vi "HFRR ADV v016 new software.vi"() -> ()   [LabVIEW 2025] (continued)
    n1463 = formula code="// Dynamic Parameterized Linear Interpolation Node\n// Inputs: vpp_val, voltages (Array), distances (Array)\n// Outputs: stroke\n\nint i = 0;\nint segments = 11; // 12 points make 11 interpolation segments\n\n// 1. Lower Boundary Clamp\nif (vpp_val <= voltages[0]) {\n    stroke = distances[0];\n}\n// 2. Upper Boundary Clamp\nelse if (vpp_val >= voltages[segments]) {\n    stroke = distances[segments];\n}\n// 3. Dynamic Segment Search Loop\nelse {\n    stroke = distances[0]; // Fallback baseline\n    for (i = 0; i < segments; i++) {\n        if (vpp_val >= voltages[i] && vpp_val <= voltages[i+1]) {\n            // Standard linear interpolation formula using array lookups\n            stroke = distances[i] + (vpp_val - voltages[i]) * (distances[i+1] - distances[i]) / (voltages[i+1] - voltages[i]);\n            break; // Segment found, safely exit the loop\n        }\n    }\n}"("vpp_val"=w1655, "voltages"="calibration values", "distances"="STROKE") -> ("stroke"=→"LVDT STROKE":dbl)
    n1464 = local read "Calibration Tare Value"() -> (w1659:dbl)
    n1465 = local read "Calibration Tare"() -> (w1657:bool)
    n1466 = Subtract(x=w1654, y=w1659) -> (x-y=→"LVDT STROKE  Calibration":dbl)
    n1467 = case shown="True" w1657 {
      selector: w1657 -> [_ w1665]
      tunnel: w1654 -> [_ w1666]
      frame False {
      }
      frame True {
        n1468 = Not(x=w1665) -> (.not. x?=w1664:bool)
        n1469 = local write "Calibration Tare"(w1664) -> ()
        "Calibration Tare Value" <- w1666
      }
    }
    n1470 = local read "Quit"() -> (w1663:bool)
  }
  n1471 = while {
    stop <- w1686 stop-if-true
    n1472 = call <vilib>:"High Resolution Polling Wait.vi"("seconds to wait"=0.02) -> ()  [unwired: 10 in, 1 out]
    n1473 = local read "Due read"() -> (w1684:string)
    n1474 = Spreadsheet String To Array(delimiter (Tab)=";", format string="", spreadsheet string=w1684, array type (2D Dbl)=string[] []) -> (array=w1681:string[])
    n1475 = Fract/Exp String To Number(string=w1681) -> (number=w1680:dbl[])  [unwired: 3 in, 1 out]
    n1476 = Index Array(array=w1680) -> (element #1=→"Sample Temperature":dbl, element #2=→"Target Sample Temperature":dbl, element #3=→"Current Duty Cycle":dbl, element #4=→"Ambient Temperature":dbl, element #5=→"Dac Status":dbl, element #6=→"Vpp":dbl, element #7=→"Active Error Code":dbl, element #8=→"Kp":dbl, element #9=→"Ki":dbl, element #10=→"Kd":dbl, element #11=→"SampleRaw":dbl, element #12=→"AmbRaw":dbl)  [unwired: 12 in]
    n1477 = local read "Quit"() -> (w1686:bool)
  }
  n1478 = while {
    shift-right: [w1700] -> w37
    shift-left: _ -> [w1691]
    shift-right: [w1699] -> w36
    shift-left: errorcluster {"status"=FALSE, "code"=0, "source"="Init"} ("error out") -> [w1693]
    tunnel: [w1688] -> w41
    tunnel: [w1698] -> _
    i -> [w1698]
    stop <- w1688 stop-if-true
    n1479 = local read "Com Port 2"() -> (w1692:refnum<visa-resource-name>)
    n1480 = local read "Port 2a"() -> (w1694:bool)
    n1481 = Unbundle(w1693) -> ("status"=→"Port 4":bool)  [unwired: 2 out]
    n1482 = call <vilib>:"High Resolution Polling Wait.vi"("seconds to wait"=0.02) -> ()  [unwired: 10 in, 1 out]
    n1483 = local read "Port 4"() -> (w1695:bool)
    n1484 = Not Equal?(x=w1692, y=w1691) -> (x != y?=w1690:bool)
    n1485 = Or(x=w1695, y=w1694) -> (x .or. y?=w1697:bool)
    n1486 = case shown="False" w1697 {
      frame False {
        w1703 = TRUE ("Visible")
        n1487 = property on="Port 2a" class="Bool (strict)"("Visible"=w1703) -> ()  [unwired: 2 in, 2 out]
        n1488 = property on="Port 4" class="Bool (strict)"("Visible"=w1703) -> ()  [unwired: 2 in, 2 out]
      }
      frame True {
        w1704 = TRUE ("Visible")
        n1489 = property on="Port 2a" class="Bool (strict)"("Visible"=w1704) -> ()  [unwired: 2 in, 2 out]
        n1490 = property on="Port 4" class="Bool (strict)"("Visible"=w1704) -> ()  [unwired: 2 in, 2 out]
      }
    }
    n1491 = case shown="True" w1690 {
      tunnel: [w1701 errorcluster {"status"=TRUE, "code"=0, "source"="Init"} ("error out")] -> w1689
      tunnel: w1693 -> [w1701 _]
      frame False {
      }
      frame True {
      }
    }
    n1492 = case shown="No Error" w1689 {
      selector: w1689 -> [w1717 w1748]
      tunnel: [w1710 w1753] -> w1700
      tunnel: [w1718 w1746] -> w1699
      tunnel: w1691 -> [w1719 w1751]
      frame No Error {
        n1493 = property class="Instr" props=["Serial Settings:Number of Bytes at Serial Port"](reference=w1719, error in=w1717) -> (reference out=w1711:refnum<visa-resource-name>, error out=w1716:errorcluster)  [unwired: 1 out]
        n1494 = while {
          tunnel: [w1727] -> w1712
          tunnel: [w1726] -> w1713
          tunnel: w1716 -> [w1725]
          tunnel: w1711 -> [w1724]
          tunnel: [w1723] -> _
          i -> [w1723]
          stop <- TRUE stop-if-true
          n1495 = property class="Instr" props=["Serial Settings:Number of Bytes at Serial Port"](reference=w1724, error in=w1725) -> (reference out=w1729:refnum<visa-resource-name>, error out=w1728:errorcluster)  [unwired: 1 out]
          n1496 = VISA Read(VISA resource name=w1729, byte count=u32 1000, error in (no error)=w1728) -> (VISA resource name out=w1726:refnum<visa-resource-name>, read buffer=→"Due read":string, error out=w1727:errorcluster)  [unwired: 1 out]
        }
        n1497 = local read "Command"() -> (w1709:string)
        n1498 = call <vilib>:"Trim Whitespace.vi"("string"=w1709) -> ("trimmed string"=w1708:string)  [unwired: 1 in]
        n1499 = Not Equal?(x=w1708, y="") -> (x != y?=w1714:bool)
        n1500 = VISA Flush I/O Buffer(VISA resource name=w1713) -> (VISA resource name out=w1706:refnum<visa-resource-name>, error out=→"error out 10":errorcluster)  [unwired: 2 in]
        n1501 = case shown="True" w1714 {
          tunnel: w1706 -> [w1731 w1736]
          tunnel: [w1731 w1740] -> w1710
          tunnel: w1712 -> [w1730 w1735]
          tunnel: [w1730 w1738] -> w1718
          tunnel: w1708 -> [_ w1734]
          tunnel: [_ w1737] -> _
          frame False {
            # "DATA  WRITE LOOP"
          }
          frame True {
            n1502 = Concatenate Strings(w1734, "\r\n") -> (w1733:string)
            n1503 = VISA Write(VISA resource name=w1736, write buffer=w1733, error in (no error)=w1735) -> (VISA resource name out=w1740:refnum<visa-resource-name>, return count=w1737:u32, error out=w1739:errorcluster)
            n1504 = flat-sequence {
              tunnel: w1739 -> [w1742]
              tunnel: [w1742] -> w1738
              frame #0 {
                n1505 = local write "Command"("" ("Command")) -> ()
                n1506 = Wait (ms)(milliseconds to wait=u32 5) -> ()  [unwired: 1 out]
              }
            }
          }
        }
        "Port 2a" <- TRUE ("Port 2a")
      }
      frame Error {
        w1759 = u16 0 items=["None", "XON/XOFF", "RTS/CTS", "XON/XOFF & RTS/CTS", "DTR/DSR", "XON/XOFF & DTR/DSR"] ("flow control (0:none)  2")
        w1757 = u16 10 items=["1.0"=10, "1.5"=15, "2.0"=20] ("stop bits 2")
        w1755 = u16 0 items=["None", "Odd", "Even", "Mark", "Space"] ("parity 2")
        w1756 = u32 10000  # timeout (10sec)
        n1507 = VISA Clear(VISA resource name=w1751, error in (no error)=w1748) -> (VISA resource name out=w1750:refnum<visa-resource-name>, error out=w1749:errorcluster)
        n1508 = VISA Close(VISA resource name=w1750, error in (no error)=w1749) -> (error out=w1752:errorcluster)
        n1509 = call <vilib>:"Clear Errors.vi"("error in (no error)"=w1752) -> ()  [unwired: 5 in, 2 out]
        n1510 = local write "Port 2a"(FALSE ("Port 2a")) -> ()
        n1511 = local read "Com Port 2"() -> (w1745:refnum<visa-resource-name>)
        "visa due" <- w1745
        n1512 = call-poly "VISA Configure Serial Port"("VISA resource name"=w1745, "timeout (10sec)"=w1756, "baud rate (9600)"=u32 250000 ("baud rate  2"), "data bits (8)"=u16 8 ("data bits  2"), "parity (0:none)"=w1755, "stop bits (10: 1 bit)"=w1757, "flow control (0:none)"=w1759) -> ("VISA resource name out"=w1760:refnum<visa-resource-name>, "error out"=w1761:errorcluster)  [unwired: 7 in]
        n1513 = flat-sequence {
          tunnel: w1760 -> [w1763]
          tunnel: w1761 -> [w1762]
          tunnel: [w1763] -> w1753
          tunnel: [w1762] -> w1746
          frame #0 {
            n1514 = Wait (ms)(milliseconds to wait=u32 50) -> ()  [unwired: 1 out]
          }
        }
        "Residual Due" <- ""
        "Port 2 Error" <- w1746
      }
    }
    n1515 = local read "Quit"() -> (w1688:bool)
    "Error Due" <- w1693
  }
  n1516 = local write "FRICVALZ"(0.0 ("FRICVALZ")) -> ()
  n1517 = property on="RUN" class="Bool (strict)"("Visible"=TRUE) -> ()  [unwired: 2 in, 2 out]
  n1518 = while {
    tunnel: [w1780] -> _
    tunnel: [w1765] -> w54
    i -> [w1780]
    stop <- w1765 stop-if-true
    n1519 = local read "conststatus"() -> (w1769:dbl)
    n1520 = local read "Main Tab"() -> (w1767:T2)
    n1521 = local read "EDIT"() -> (w1786:bool)
    n1522 = local read "Rate"() -> (w1785:dbl)
    n1523 = case shown="True" w1786 {
      tunnel: [FALSE TRUE] -> w1772
      frame False {
      }
      frame True {
      }
    }
    n1524 = property on="Time slide" class="Slide (strict)"("Scale.Range:Maximum"=2500.0) -> ()  [unwired: 2 in, 2 out]
    n1525 = Equal?(x=w1767, y=T27."About" ("Main Tab")) -> (x = y?=w1778:bool)
    n1526 = Equal?(x=w1769, y=0.0) -> (x = y?=w1770:bool)
    n1527 = Divide(x=1.0, y=w1785) -> (x/y=w1781:dbl)
    "Time 2" <- w1781
    n1528 = case shown="True" w1770 {
      frame False {
      }
      frame True {
        # "C:\\WinDucom\\calibrate WO 2391.dcf"
        n1529 = local write "Lan flag"(22) -> ()
        n1530 = local write "conststatus"(10.0 ("rpm value : 2")) -> ()
        n1531 = String To Path(string="C:\\LAB-IQ\\calibrate WO 2465.dcf") -> (path=w1792:path)
        n1532 = Open/Create/Replace File "Open File"(file path (use dialog)=w1792) -> (refnum out=w1790:refnum<file>)  [unwired: 5 in, 2 out]
        n1533 = for {
          N: 23 -> [_]
          tunnel: w1790 -> [w1801]
          i -> [w1795]
          (unwired) TRUE ("line mode (F)")
          n1534 = Read from Text File "Read File"(file (use dialog)=w1801) -> (text=w1800:string)  [unwired: 3 in, 3 out]
          n1535 = Match Pattern(string=w1800, regular expression="]") -> (after substring=w1798:string)  [unwired: 1 in, 3 out]
          n1536 = String Subset(string=w1800, offset (0)=5, length (rest)=10 ("length (rest)")) -> (substring=w1793:string)
          n1537 = Fract/Exp String To Number(string=w1793) -> (number=w1794:dbl)  [unwired: 3 in, 1 out]
          n1538 = Match Pattern(string=w1798, regular expression="-") -> (before substring=w1796:string)  [unwired: 1 in, 3 out]
          n1539 = case shown="19" w1795 {
            tunnel: w1794 -> [w1804 w1805 w1806 w1807 _ _ _ w1812 w1813 _ w1814 w1815 w1816 w1817 w1818 w1819 _ w1820 w1821 _ _ _ _ _]
            tunnel: w1796 -> [_ _ _ _ w1808 w1809 w1810 _ _ _ _ _ _ _ _ _ _ _ _ w1822 w1823 w1824 w1825 _]
            frame 0 {
              n1540 = local write "FRIC. FORCE :"(w1804) -> ()
            }
            frame 1 {
              n1541 = local write "TEMPERATURE :"(w1805) -> ()
            }
            frame 2 {
              n1542 = local write "HUMIDITY:"(w1806) -> ()
            }
            frame 3 {
              n1543 = local write "AIR TEMPERATURE :"(w1807) -> ()
            }
            frame 4 {
              n1544 = local write "Com Port 1"(w1808) -> ()
            }
            frame 5 {
              n1545 = local write "Com Port 2"(w1809) -> ()
              n1546 = local write "visa due"(w1809) -> ()
            }
            frame 6 {
              n1547 = String To Path(string=w1810) -> (path=w1811:path)
              n1548 = local write "File Path"(w1811) -> ()
              "String" <- w1810
            }
            frame 7 {
              n1549 = local write "DISPLACEMENT :"(w1812) -> ()
            }
            frame 8 {
              n1550 = local write "STROKE GAIN :"(w1813) -> ()
            }
            frame 9 {
            }
            frame 10 {
              n1551 = local write "Language Selection"(w1814) -> ()
            }
            frame 11 {
              n1552 = local write "CH-POWER +"(w1815) -> ()
            }
            frame 12 {
              n1553 = local write "CH-POWER -"(w1816) -> ()
            }
            frame 13 {
              n1554 = local write "CH-HEATER"(w1817) -> ()
            }
            frame 14 {
              n1555 = local write "CH-HUMIDITY WET"(w1818) -> ()
            }
            frame 15 {
              n1556 = local write "CH-HUMIDITY DRY"(w1819) -> ()
            }
            frame 16 {
            }
            frame 17 {
              n1557 = local write "AIR TEMP INTERCEPT:"(w1820) -> ()
            }
            frame 18 {
              n1558 = local write "TEMP INTERCEPT:"(w1821) -> ()
            }
            frame 21 {
              n1559 = local write "S.NO"(w1822) -> ()
            }
            frame 22 {
              n1560 = local write "Com Port 3"(w1823) -> ()
            }
            frame 20 {
              n1561 = local write "Camera Port :"(w1824) -> ()
            }
            frame 19 {
              n1562 = local write "C3 :"(w1825) -> ()
            }
            frame 23, Default {
            }
          }
        }
      }
    }
    n1563 = Select(t=u32 2500 ("milliseconds to wait"), s=w1778, f=u32 500 ("milliseconds to wait")) -> (s? t:f=w1776:u32)
    n1564 = Multiply(x=w1781, y=w1776) -> (x*y=w1783:dbl)
    n1565 = property on="Time slide" class="Slide (strict)"("Visible"=w1772) -> ()  [unwired: 2 in, 2 out]
    n1566 = call "Elapsed Time2"("Time Target (s)"=w1783, "Auto Reset"=TRUE) -> ("Time has Elapsed"=w1773:bool)  [unwired: 10 in, 7 out]
    n1567 = case shown="True" w1773 {
      frame False {
      }
      frame True {
        n1568 = stacked-sequence {
          frame #0 {
            # "DATA PROCESSING"
            # "115 mV/N"
            n1569 = local read "Sample Temperature"() -> (w1828:dbl)
            n1570 = local read "RH Numeric:"() -> (w1835:dbl)
            n1571 = local read "HUMIDITY:"() -> (w1836:dbl)
            n1572 = local read "FRICVALZ"() -> (w1847:dbl)
            n1573 = local read "Friction"() -> (w1831:dbl)
            n1574 = Multiply(x=w1835, y=w1836) -> (x*y=→"Humidity ( %RH )" →"Hum" →"Hum 2":dbl)
            n1575 = call <vilib>:"Mean PtByPt.vi"("x"=w1828, "sample length"=100) -> ("mean"=w1827:dbl)  [unwired: 2 in, 1 out]
            "TEMP 2" <- w1827
            "TEMP 3" <- w1827
            n1576 = Subtract(x=w1831, y=w1847) -> (x-y=w1842:dbl)
            "FF 2" <- w1842
            "FF 4" <- w1842
            n1577 = local read "Ambient Temperature"() -> (→"AIR TEMP":dbl)
            n1578 = local read "TEMP"() -> (w1846:dbl)
            n1579 = local write "FF 3"(w1842) -> ()
            n1580 = Compound Arithmetic op=OR("FRICVALZ 4", "FRICVALZ 3", "FRICVALZ 2") -> (w1838:bool)
            n1581 = case shown="True" w1838 {
              tunnel: w1831 -> [_ w1853]
              frame False {
              }
              frame True {
                w1852 = FALSE ("FRICVALZ")
                n1582 = local write "FRICVALZ 3"(w1852) -> ()
                n1583 = local write "FRICVALZ 2"(w1852) -> ()
                n1584 = local write "FRICVALZ 4"(w1852) -> ()
                "FRICVALZ" <- w1853
              }
            }
            n1585 = Not A Number/Path/Refnum?(number/path/refnum=w1846) -> (NaN/Path/Refnum?=w1845:bool)
            n1586 = Not A Number/Path/Refnum?(number/path/refnum=w1842) -> (NaN/Path/Refnum?=w1844:bool)
            n1587 = Divide(x=w1842, y=1.96) -> (x/y=w1839:dbl)
            n1588 = Compound Arithmetic op=OR(w1845, w1844) -> (w1843:bool)
            n1589 = Not A Number/Path/Refnum?(number/path/refnum=w1839) -> (NaN/Path/Refnum?=w1840:bool)
            n1590 = case shown="True" w1843 {
              frame False {
              }
              frame True {
                n1591 = local write "TEMP"(0.0 ("TEMP")) -> ()
                n1592 = local write "FF 2"(0.0 ("FF 2")) -> ()
                n1593 = local write "reinit"(TRUE ("reinit")) -> ()
              }
            }
            n1594 = local write "TEMP"(w1827) -> ()
            n1595 = Select(t=0.0, s=w1840, f=w1839) -> (s? t:f=w1830:dbl)
            "COF 2" <- w1830
            n1596 = local write "COF 3"(w1830) -> ()
          }
        }
      }
    }
    n1597 = Wait (ms)(milliseconds to wait=u32 50) -> ()  [unwired: 1 out]
    n1598 = local read "Quit"() -> (w1765:bool)
    "Rate" <- 2500.0 ("No of Samples")
  }
  n1599 = while {
    tunnel: w57 -> [_]
    tunnel: [w1880] -> _
    tunnel: [w1856] -> w56
    i -> [w1880]
    stop <- w1856 stop-if-true
    # "C:\\LAB-IQ-NXT\\Scar View.exe"
    n1600 = local read "OK Button 16"() -> (w1869:bool)
    n1601 = local read "Main Tab"() -> (w1862:T2)
    n1602 = local read "service 3"() -> (w1863:bool)
    n1603 = local read "OPEN 6"() -> (w1865:bool)
    n1604 = local read "EDIT 2"() -> (w1867:bool)
    n1605 = flat-sequence {
      frame #0 {
        n1606 = local read "SAVE 2"() -> (w2482:bool)
        n1607 = stacked-sequence {
          frame #0 {
            n1608 = local read "EDIT"() -> (w2536:bool)
            n1609 = case shown="True" w2536 {
              tunnel: [u8 2 ("Disabled") u8 0 ("Disabled")] -> _
              frame False {
                w2538 = FALSE
                n1610 = local write "Password"("") -> ()
                n1611 = property on="SrvM CP" class="Bool (strict)"("Visible"=w2538) -> ()  [unwired: 2 in, 2 out]
                n1612 = property on="message" class="Str"("Visible"=w2538) -> ()  [unwired: 2 in, 2 out]
                n1613 = local write "x = y?"(w2538) -> ()
                n1614 = property on="Password" class="Str"("Visible"=w2538) -> ()  [unwired: 2 in, 2 out]
                n1615 = property on="ENTER THE NEW PASSWORD" class="Str"("Visible"=w2538) -> ()  [unwired: 2 in, 2 out]
                n1616 = property on="ENTER CURRENT PASSWORD" class="Str"("Visible"=w2538) -> ()  [unwired: 2 in, 2 out]
                n1617 = local write "SrvM CP"(w2538) -> ()
              }
              frame True {
                w2541 = TRUE
                n1618 = property on="SrvM CP" class="Bool (strict)"("Visible"=w2541) -> ()  [unwired: 2 in, 2 out]
                n1619 = property on="Password" class="Str"("Visible"=w2541) -> ()  [unwired: 2 in, 2 out]
              }
            }
            "dipl pwd" <- "@143$\n" ("dipl pwd")
          }
          frame #1 {
            # "Gain password"
            n1620 = String To Byte Array(string="ENTER CURRENT PASSWORD") -> (unsigned byte array=w2546:u8[])
            n1621 = Search 1D Array(1D array=w2546, element=u8 10) -> (index of element=w2549:i32)  [unwired: 1 in]
            n1622 = Index Array(array=w2546, index=w2549) -> (element=w2545:u8)
            n1623 = Equal?(x=w2545, y=10) -> (x = y?=w2543:bool)
            n1624 = case shown="True" w2543 {
              frame False {
                n1625 = property on="ENTER THE NEW PASSWORD" class="Str"("Visible"=FALSE) -> ()  [unwired: 2 in, 2 out]
              }
              frame True {
                # "password"
                # "change password logic"
                n1626 = local read "ENTER CURRENT PASSWORD"() -> (w2562:string)
                n1627 = local read "dipl pwd"() -> (w2556:string)
                n1628 = String To Byte Array(string=w2562) -> (unsigned byte array=w2564:u8[])
                n1629 = String To Byte Array(string=w2556) -> (unsigned byte array=w2557:u8[])
                n1630 = Array Size(array=w2564) -> (size(s)=w2561:i32)
                n1631 = Array Size(array=w2557) -> (size(s)=w2559:i32)
                n1632 = for {
                  N: w2561 -> [_]
                  tunnel: w2564 -> [w2588]
                  tunnel: [w2586] -> w2565 mode=indexing
                  tunnel: w2561 -> [w2580]
                  i -> [w2581]
                  n1633 = Decrement(x=w2580) -> (x-1=w2578:i32)
                  n1634 = Equal?(x=w2581, y=w2578) -> (x = y?=w2579:bool)
                  n1635 = Index Array(array=w2588, index=w2581) -> (element=w2582:u8)
                  n1636 = Number To Decimal String(number=w2582) -> (decimal integer string=w2587:string)  [unwired: 1 in]
                  n1637 = Select(t="", s=w2579, f="\r") -> (s? t:f=w2584:string)
                  n1638 = Concatenate Strings(w2587, w2584) -> (w2586:string)
                }
                n1639 = for {
                  N: w2559 -> [_]
                  tunnel: w2557 -> [w2576]
                  tunnel: [w2574] -> w2558 mode=indexing
                  tunnel: w2559 -> [w2571]
                  i -> [w2572]
                  n1640 = Decrement(x=w2571) -> (x-1=w2570:i32)
                  n1641 = Equal?(x=w2572, y=w2570) -> (x = y?=w2569:bool)
                  n1642 = Index Array(array=w2576, index=w2572) -> (element=w2575:u8)
                  n1643 = Number To Decimal String(number=w2575) -> (decimal integer string=w2573:string)  [unwired: 1 in]
                  n1644 = Select(t="", s=w2569, f="\r") -> (s? t:f=w2566:string)
                  n1645 = Concatenate Strings(w2573, w2566) -> (w2574:string)
                }
                n1646 = local read "string"() -> (w2563:string)
                n1647 = Concatenate Strings(w2558) -> (w2552:string)
                n1648 = Concatenate Strings(w2563) -> (w2560:string)
                n1649 = Concatenate Strings(w2565) -> (w2553:string)
                n1650 = Equal?(x=w2553, y=w2560) -> (x = y?=w2555:bool)
                n1651 = Equal?(x=w2553, y=w2552) -> (x = y?=w2551:bool)
                n1652 = Or(x=w2555, y=w2551) -> (x .or. y?=w2554:bool)
                n1653 = case shown="True" w2554 {
                  frame False {
                  }
                  frame True {
                    n1654 = property on="ENTER THE NEW PASSWORD" class="Str"("Visible"=TRUE) -> ()  [unwired: 2 in, 2 out]
                  }
                }
              }
            }
          }
          frame #2 {
            n1655 = String To Byte Array(string="ENTER THE NEW PASSWORD") -> (unsigned byte array=w2591:u8[])
            n1656 = Search 1D Array(1D array=w2591, element=u8 10) -> (index of element=w2595:i32)  [unwired: 1 in]
            n1657 = Index Array(array=w2591, index=w2595) -> (element=w2593:u8)
            n1658 = Equal?(x=w2593, y=10) -> (x = y?=w2590:bool)
            n1659 = case shown="False" w2590 {
              frame False {
              }
              frame True {
                n1660 = local write "EDIT"(FALSE) -> ()
                n1661 = local write "SrvM CP"(FALSE) -> ()
                n1662 = local read "ENTER THE NEW PASSWORD"() -> (w2598:string)
                n1663 = String To Byte Array(string=w2598) -> (unsigned byte array=w2603:u8[])
                n1664 = Array Size(array=w2603) -> (size(s)=w2600:i32)
                n1665 = for {
                  N: w2600 -> [_]
                  tunnel: w2603 -> [w2616]
                  tunnel: [w2613] -> w2605 mode=indexing
                  tunnel: w2600 -> [w2608]
                  i -> [w2606]
                  n1666 = Decrement(x=w2608) -> (x-1=w2609:i32)
                  n1667 = Equal?(x=w2606, y=w2609) -> (x = y?=w2610:bool)
                  n1668 = Index Array(array=w2616, index=w2606) -> (element=w2615:u8)
                  n1669 = Number To Decimal String(number=w2615) -> (decimal integer string=w2614:string)  [unwired: 1 in]
                  n1670 = Select(t="", s=w2610, f="\r") -> (s? t:f=w2607:string)
                  n1671 = Concatenate Strings(w2614, w2607) -> (w2613:string)
                }
                n1672 = local read "file path"() -> (w2597:path)
                n1673 = Concatenate Strings(w2605) -> (w2599:string)
                n1674 = Delete(path (use dialog)=w2597) -> (deleted path=w2601:path)  [unwired: 4 in, 2 out]
                n1675 = call <vilib>:"Write Characters To File.vi"("append to file? (new file:F)"=FALSE, "character string"=w2599, "file path (dialog if empty)"=w2601) -> ()  [unwired: 2 in, 1 out]
              }
            }
          }
          frame #3 {
            n1676 = case shown="True" "SrvM CP" {
              frame False {
                w2619 = ""
                n1677 = local write "ENTER CURRENT PASSWORD"(w2619) -> ()
                n1678 = local write "ENTER THE NEW PASSWORD"(w2619) -> ()
                n1679 = property on="ENTER CURRENT PASSWORD" class="Str"("Visible"=FALSE) -> ()  [unwired: 2 in, 2 out]
              }
              frame True {
                n1680 = property on="ENTER THE NEW PASSWORD" class="Str"() -> ("Visible"=w2620:bool)  [unwired: 2 in, 2 out]
                n1681 = Not(x=w2620) -> (.not. x?=w2621:bool)
                n1682 = property on="ENTER CURRENT PASSWORD" class="Str"("Visible"=w2621) -> ()  [unwired: 2 in, 2 out]
              }
            }
          }
          frame #4 {
            n1683 = String To Byte Array(string="Password") -> (unsigned byte array=w2628:u8[])
            n1684 = Search 1D Array(1D array=w2628, element=u8 10) -> (index of element=w2626:i32)  [unwired: 1 in]
            n1685 = Index Array(array=w2628, index=w2626) -> (element=w2627:u8)
            n1686 = Equal?(x=w2627, y=10) -> (x = y?=w2623:bool)
            n1687 = case shown="True" w2623 {
              frame False {
              }
              frame True {
                # "password"
                # "password"
                n1688 = local read "Password"() -> (w2641:string)
                n1689 = String To Byte Array(string=w2641) -> (unsigned byte array=w2644:u8[])
                n1690 = String To Byte Array(string="@143$\n") -> (unsigned byte array=w2630:u8[])
                n1691 = Array Size(array=w2644) -> (size(s)=w2639:i32)
                n1692 = Array Size(array=w2630) -> (size(s)=w2635:i32)
                n1693 = for {
                  N: w2639 -> [_]
                  tunnel: w2644 -> [w2678]
                  tunnel: [w2676] -> w2645 mode=indexing
                  tunnel: w2639 -> [w2673]
                  i -> [w2674]
                  n1694 = Decrement(x=w2673) -> (x-1=w2672:i32)
                  n1695 = Index Array(array=w2678, index=w2674) -> (element=w2677:u8)
                  n1696 = Equal?(x=w2674, y=w2672) -> (x = y?=w2671:bool)
                  n1697 = Number To Decimal String(number=w2677) -> (decimal integer string=w2675:string)  [unwired: 1 in]
                  n1698 = Select(t="", s=w2671, f="\r") -> (s? t:f=w2668:string)
                  n1699 = Concatenate Strings(w2675, w2668) -> (w2676:string)
                }
                n1700 = for {
                  N: w2635 -> [_]
                  tunnel: w2630 -> [w2689]
                  tunnel: [w2687] -> w2633 mode=indexing
                  tunnel: w2635 -> [w2684]
                  i -> [w2685]
                  n1701 = Decrement(x=w2684) -> (x-1=w2683:i32)
                  n1702 = Index Array(array=w2689, index=w2685) -> (element=w2688:u8)
                  n1703 = Equal?(x=w2685, y=w2683) -> (x = y?=w2682:bool)
                  n1704 = Number To Decimal String(number=w2688) -> (decimal integer string=w2686:string)  [unwired: 1 in]
                  n1705 = Select(t="", s=w2682, f="\r") -> (s? t:f=w2679:string)
                  n1706 = Concatenate Strings(w2686, w2679) -> (w2687:string)
                }
                n1707 = local read "file path"() -> (w2629:path)
                n1708 = call <vilib>:"Read Characters From File.vi"("file path (dialog if empty)"=w2629) -> ("character string"=w2643:string)  [unwired: 5 in, 3 out]
                "string" <- w2643
                n1709 = flat-sequence {
                  tunnel: [w2646] -> w2640
                  frame #0 {
                    w2646 = ""
                    n1710 = local write "Password"(w2646) -> ()
                  }
                }
                n1711 = Concatenate Strings(w2633) -> (w2634:string)
                n1712 = Concatenate Strings(w2643) -> (w2642:string)
                n1713 = Concatenate Strings(w2645) -> (w2637:string)
                n1714 = Equal?(x=w2637, y=w2642) -> (x = y?=w2632:bool)
                n1715 = Equal?(x=w2637, y=w2634) -> (x = y?=w2638:bool)
                n1716 = Or(x=w2632, y=w2638) -> (x .or. y?=w2631:bool)
                "x = y?" <- w2631
                n1717 = case shown="True" w2631 {
                  selector: w2631 -> [w2648 _]
                  tunnel: w2640 -> [_ _]
                  frame False {
                    n1718 = And(x=w2648, y=TRUE ("Visible")) -> (x .and. y?=w2649:bool)
                    n1719 = property on="message" class="Str"("Visible"=w2649) -> ()  [unwired: 2 in, 2 out]
                  }
                  frame True {
                    n1720 = control-ref of="This VI"() -> (w2660:refnum<vi>)
                    n1721 = property class="VI"(reference=w2660) -> (reference out=w2651:refnum<vi>, error out=w2655:errorcluster, "Panel"=w2659:refnum<vi>)  [unwired: 1 in]
                    n1722 = property on="message" class="Str"("Visible"=FALSE) -> ()  [unwired: 2 in, 2 out]
                    n1723 = property class="Pnl"(reference=w2659, error in=w2655) -> (reference out=w2653:refnum<vi>, error out=w2656:errorcluster, "Panes[]"=w2658:refnum<vi>[])
                    n1724 = for {
                      tunnel: w2658 -> [w2667] mode=indexing
                      tunnel: T21."Always On" ("Horizontal Scrollbar Visibility") -> [w2666]
                      tunnel: w2656 -> [w2663]
                      tunnel: [w2662] -> w2654
                      n1725 = property class="Pane"(reference=w2667, error in=w2663, "HorizScrollbarVisibility"=w2666) -> (reference out=w2664:refnum<vi>, error out=w2665:errorcluster)
                      n1726 = Close Reference(reference=w2664, error in (no error)=w2665) -> (error out=w2662:errorcluster)
                    }
                    n1727 = Close Reference(reference=w2653, error in (no error)=w2654) -> (error out=w2652:errorcluster)
                    n1728 = Close Reference(reference=w2651, error in (no error)=w2652) -> (error out=→"error out 6":errorcluster)
                  }
                }
              }
            }
          }
        }
        n1729 = local read "x = y?"() -> (w2488:bool)
        n1730 = local read "HUMIDITY: 2"() -> (w2490:dbl)
        n1731 = local read "HUMIDITY:"() -> (w2489:dbl)
        n1732 = property on="Port 2 Error" class="Clust (strict)"("Visible"="EDIT") -> ()  [unwired: 2 in, 2 out]
        n1733 = property on="Port 1 Error" class="Clust (strict)"("Visible"="EDIT") -> ()  [unwired: 2 in, 2 out]
        n1734 = case shown="True" "SrvM CP 2" {
          frame False {
          }
          frame True {
            n1735 = local write "SrvM CP 2"(FALSE ("SrvM CP 2")) -> ()
            n1736 = local read "HUMIDITY: 2"() -> (w2529:dbl)
            n1737 = local read "TEMP INTERCEPT: 2"() -> (w2528:dbl)
            n1738 = local read "DISPLACEMENT : 4"() -> (w2532:dbl)
            n1739 = local read "TEMPERATURE : 2"() -> (w2531:dbl)
            n1740 = local read "STROKE GAIN : 2"() -> (w2533:dbl)
            n1741 = local read "FRIC. FORCE : 2"() -> (w2534:dbl)
            n1742 = local read "AIR TEMP INTERCEPT: 2"() -> (w2527:dbl)
            n1743 = local read "AIR TEMPERATURE : 2"() -> (w2530:dbl)
            n1744 = local write "HUMIDITY:"(w2529) -> ()
            n1745 = local write "AIR TEMP INTERCEPT:"(w2528) -> ()
            n1746 = local write "TEMPERATURE :"(w2531) -> ()
            n1747 = local write "FRIC. FORCE :"(w2534) -> ()
            n1748 = local write "STROKE GAIN :"(w2533) -> ()
            n1749 = local write "DISPLACEMENT :"(w2532) -> ()
            n1750 = local write "AIR TEMPERATURE :"(w2530) -> ()
            n1751 = local write "TEMP INTERCEPT:"(w2527) -> ()
          }
        }
        n1752 = Or(x="SAVE", y=w2482) -> (x .or. y?=w2483:bool)
        n1753 = And(x="EDIT", y=w2488) -> (x .and. y?=w2486:bool)
        n1754 = local read "DISPLACEMENT : 4"() -> (w2499:dbl)
        n1755 = local read "TEMPERATURE : 2"() -> (w2497:dbl)
        n1756 = local read "STROKE GAIN : 2"() -> (w2503:dbl)
        n1757 = local read "DISPLACEMENT :"() -> (w2498:dbl)
        n1758 = local read "FRIC. FORCE : 2"() -> (w2506:dbl)
        n1759 = local read "TEMPERATURE :"() -> (w2495:dbl)
        n1760 = local read "STROKE GAIN :"() -> (w2502:dbl)
        n1761 = local read "FRIC. FORCE :"() -> (w2505:dbl)
        n1762 = case shown="True" w2486 {
          tunnel: [u8 2 ("Disabled") u8 0 ("Disabled")] -> w2485
          tunnel: [w2850 TRUE ("Visible")] -> w2484
          frame False {
            w2850 = FALSE ("Visible")
            n1763 = local write "EDIT 2"(w2850) -> ()
          }
          frame True {
          }
        }
        n1764 = case shown="True" w2483 {
          frame False {
          }
          frame True {
            n1765 = stacked-sequence {
              seq-local: [w2698 _ _] -> [_ w2845 _]
              frame #0 {
                (unwired) i16 5 ("precision (6)")
                # "[CH1]    - FF\n[CH2]   - TEMPERATURE\n[CH3]    - Humidity\n[CH4]    - AIR TEMP\n[CH5]\\- Visa Uno\n[CH6] \\- Visa Due\n[CH7]  \\- file path\n[CH8]   - Displacement Gain\n[CHA]   - Stroke Gain\n[CHB]   - Stroke PID Gain\n[CHC]   -Language Selection\n[CHD]   -Power +\n[CHE]   -Power_\n[CHF]   -Heater\n[CHG]   -Humidity Wet\n[CHH]   -Humidity Dry\n[CHI]   -Integral Time"
                n1766 = local read "Language Selection"() -> (w2746:enum16{"English", "Russian"})
                n1767 = local read "CH-HUMIDITY WET"() -> (w2704:u16)
                n1768 = local read "CH-HUMIDITY DRY"() -> (w2701:u16)
                n1769 = local read "STROKE GAIN :"() -> (w2690:dbl)
                n1770 = local read "CH-POWER +"() -> (w2713:u16)
                n1771 = local read "CH-POWER -"() -> (w2710:u16)
                n1772 = local read "CH-HEATER"() -> (w2707:u16)
                n1773 = local read "AIR TEMPERATURE :"() -> (w2693:dbl)
                n1774 = local read "DISPLACEMENT :"() -> (w2691:dbl)
                n1775 = local read "TEMPERATURE :"() -> (w2694:dbl)
                n1776 = local read "FRIC. FORCE :"() -> (w2695:dbl)
                n1777 = local read "HUMIDITY:"() -> (w2692:dbl)
                n1778 = Path To String(path="File Path") -> (string=w2762:string)
                n1779 = Number To Fractional String(number=w2690, width (-)=i16 10 ("precision (6)"), precision (6)=i16 5) -> (F-format string=w2753:string)  [unwired: 1 in]
                n1780 = Number To Fractional String(number=w2746, width (-)=i16 10 ("precision (6)"), precision (6)=i16 5) -> (F-format string=w2742:string)  [unwired: 1 in]
                n1781 = Number To Fractional String(number=w2713, width (-)=i16 10 ("precision (6)"), precision (6)=i16 5) -> (F-format string=w2736:string)  [unwired: 1 in]
                n1782 = Number To Fractional String(number=w2710, width (-)=i16 10 ("precision (6)"), precision (6)=i16 5) -> (F-format string=w2733:string)  [unwired: 1 in]
                n1783 = Number To Fractional String(number=w2707, width (-)=i16 10 ("precision (6)"), precision (6)=i16 5) -> (F-format string=w2728:string)  [unwired: 1 in]
                n1784 = Number To Fractional String(number=w2704, width (-)=i16 10 ("precision (6)"), precision (6)=i16 5) -> (F-format string=w2725:string)  [unwired: 1 in]
                n1785 = Number To Fractional String(number=w2701, width (-)=i16 10 ("precision (6)"), precision (6)=i16 5) -> (F-format string=w2720:string)  [unwired: 1 in]
                n1786 = local read "Com Port 1"() -> (w2697:refnum<visa-resource-name>)
                n1787 = local read "Com Port 2"() -> (w2696:refnum<visa-resource-name>)
                n1788 = Concatenate Strings(w2762, "\\" ("string")) -> (w2761:string)
                n1789 = Number To Fractional String(number=w2695, width (-)=i16 10 ("precision (6)"), precision (6)=i16 5) -> (F-format string=w2794:string)  [unwired: 1 in]
                n1790 = Number To Fractional String(number=w2694, width (-)=i16 10 ("precision (6)"), precision (6)=i16 5) -> (F-format string=w2793:string)  [unwired: 1 in]
                n1791 = Number To Fractional String(number=w2692, width (-)=i16 10 ("precision (6)"), precision (6)=i16 5) -> (F-format string=w2787:string)  [unwired: 1 in]
                n1792 = Number To Fractional String(number=w2693, width (-)=i16 10 ("precision (6)"), precision (6)=i16 5) -> (F-format string=w2781:string)  [unwired: 1 in]
                n1793 = Number To Fractional String(number=w2691, width (-)=i16 10 ("precision (6)"), precision (6)=i16 5) -> (F-format string=w2754:string)  [unwired: 1 in]
                n1794 = Concatenate Strings("[CHA]" ("string"), w2753, "- Stroke Gain" ("string"), "\r") -> (w2747:string)
                n1795 = Concatenate Strings("[CHC]" ("string"), w2742, "-Language Selection" ("string"), "\r") -> (w2739:string)
                n1796 = Concatenate Strings("[CHD]" ("string"), w2736, "-Power +" ("string"), "\r") -> (w2718:string)
                n1797 = Concatenate Strings("[CHG]" ("string"), w2725, "-Humidity Wet" ("string"), "\r") -> (w2715:string)
                n1798 = Concatenate Strings("[CHH]" ("string"), w2720, "-Humidity Dry" ("string"), "\r") -> (w2714:string)
                n1799 = Concatenate Strings("[CH1]" ("string"), w2794, " - FF" ("string"), "\r") -> (w2792:string)
                n1800 = Concatenate Strings("[CH2]" ("string"), w2793, " - TEMPERATURE" ("string"), "\r") -> (w2791:string)
                n1801 = Concatenate Strings("[CH3]" ("string"), w2787, " - Humidity" ("string"), "\r") -> (w2784:string)
                n1802 = Concatenate Strings("[CH4]" ("string"), w2781, " - AIR TEMP" ("string"), "\r") -> (w2777:string)
                n1803 = Concatenate Strings("[CH5]" ("string"), w2697, "- Visa Uno" ("string"), "\r") -> (w2770:string)
                n1804 = Concatenate Strings("[CH6]" ("string"), w2696, "- Visa Due" ("string"), "\r") -> (w2765:string)
                n1805 = Concatenate Strings("[CH7]" ("string"), w2761, "- file path" ("string"), "\r") -> (w2764:string)
                n1806 = Concatenate Strings("[CH8]" ("string"), w2754, "- Displacement Gain" ("string"), "\r") -> (w2757:string)
                n1807 = Concatenate Strings("[CHE]" ("string"), w2733, "-Power_" ("string"), "\r") -> (w2717:string)
                n1808 = Concatenate Strings("[CHF]" ("string"), w2728, "-Heater" ("string"), "\r") -> (w2716:string)
                n1809 = Concatenate Strings(w2792, w2791, w2784, w2777, w2770, w2765, w2764, w2757, w2747, w2739, w2718, w2717, w2716, w2715, w2714) -> (w2698:string)
                "gain" <- w2698
              }
              frame #1 {
                n1810 = local read "Camera Port :"() -> (w2806:string)
                n1811 = local read "C3 :"() -> (w2814:refnum<visa-resource-name>)
                n1812 = local read "TEMP INTERCEPT:"() -> (w2815:dbl)
                n1813 = local read "AIR TEMP INTERCEPT:"() -> (w2816:dbl)
                n1814 = local read "Com Port 3"() -> (w2817:refnum<visa-resource-name>)
                n1815 = Concatenate Strings("[CH8]" ("string"), w2806, "- Visa Camera" ("string"), "\r") -> (w2805:string)
                n1816 = Concatenate Strings("[CH7]" ("string"), w2814, "- Visa Humidity" ("string"), "\r") -> (w2810:string)
                n1817 = Number To Fractional String(number=w2815, width (-)=i16 10 ("precision (6)"), precision (6)=i16 5) -> (F-format string=w2833:string)  [unwired: 1 in]
                n1818 = Concatenate Strings("[CHL]" ("string"), w2817, "- Visa humid" ("string"), "\r") -> (w2820:string)
                n1819 = Number To Fractional String(number=w2816, width (-)=i16 10 ("precision (6)"), precision (6)=i16 5) -> (F-format string=w2840:string)  [unwired: 1 in]
                n1820 = Concatenate Strings("[CHK]" ("string"), w2833, "-TEMP INTERCEPT" ("string"), "\r") -> (w2829:string)
                n1821 = Concatenate Strings("[SNO]" ("string"), "S.NO", "-" ("string"), "\r") -> (w2825:string)
                n1822 = Concatenate Strings("[CHJ]" ("string"), w2840, "-AIR TEMP INTERCEPT" ("string"), "\r") -> (w2830:string)
                n1823 = String To Path(string="C:\\LAB-IQ\\calibrate WO 2465.dcf") -> (path=w2818:path)
                n1824 = Concatenate Strings(w2845, w2830, w2829, w2825, w2820, w2810, w2805) -> (w2844:string)
                n1825 = call <vilib>:"Write Characters To File.vi"("append to file? (new file:F)"=FALSE, "character string"=w2844, "file path (dialog if empty)"=w2818) -> ()  [unwired: 2 in, 1 out]
              }
              frame #2 {
                n1826 = local write "Lan flag"(0.0 ("Lan flag")) -> ()
                n1827 = local write "conststatus"(0.0 ("rpm value : 2")) -> ()
                n1828 = local write "SAVE"(FALSE ("OK Button 14")) -> ()
                n1829 = local write "SAVE 2"(FALSE ("SAVE 2")) -> ()
              }
            }
          }
        }
        n1830 = Subtract(x=w2490, y=w2489) -> (x-y=w2491:dbl)
        n1831 = local read "AIR TEMPERATURE : 2"() -> (w2494:dbl)
        n1832 = local read "AIR TEMPERATURE :"() -> (w2493:dbl)
        n1833 = Divide(x=w2491, y=w2489) -> (x/y=w2513:dbl)
        n1834 = Subtract(x=w2506, y=w2505) -> (x-y=w2504:dbl)
        n1835 = Subtract(x=w2497, y=w2495) -> (x-y=w2496:dbl)
        n1836 = Subtract(x=w2503, y=w2502) -> (x-y=w2501:dbl)
        n1837 = Subtract(x=w2499, y=w2498) -> (x-y=w2500:dbl)
        n1838 = Subtract(x=w2494, y=w2493) -> (x-y=w2492:dbl)
        n1839 = Divide(x=w2504, y=w2505) -> (x/y=w2524:dbl)
        n1840 = Divide(x=w2496, y=w2495) -> (x/y=w2517:dbl)
        n1841 = Divide(x=w2501, y=w2502) -> (x/y=w2521:dbl)
        n1842 = Divide(x=w2500, y=w2498) -> (x/y=w2520:dbl)
        n1843 = Multiply(x=w2513, y=100.0) -> (x*y=→"HUMIDITY  Calibration Error":dbl)
        n1844 = Divide(x=w2492, y=w2493) -> (x/y=w2516:dbl)
        n1845 = Multiply(x=w2524, y=100.0) -> (x*y=→"FRIC. FORCE Calibration Error":dbl)
        n1846 = Multiply(x=w2517, y=100.0) -> (x*y=→"TEMPERATURE  Calibration Error":dbl)
        n1847 = Multiply(x=w2521, y=100.0) -> (x*y=→"STROKE Calibration Error":dbl)
        n1848 = Multiply(x=w2520, y=100.0) -> (x*y=→"DISPLACEMENT  Calibration Error":dbl)
        n1849 = property on="EDIT 2" class="Bool (strict)"("Visible"=w2484) -> ()  [unwired: 2 in, 2 out]
        n1850 = property on="SAVE" class="Bool (strict)"("Visible"=w2484) -> ()  [unwired: 2 in, 2 out]
        n1851 = property on="SrvM CP" class="Bool (strict)"("Disabled"=w2485) -> ()  [unwired: 2 in, 2 out]
        n1852 = property on="visa due" class="CmbBox"("Disabled"=w2485) -> ()  [unwired: 2 in, 2 out]
        n1853 = property on="File Path" class="Path"("Disabled"=w2485) -> ()  [unwired: 2 in, 2 out]
        n1854 = Multiply(x=w2516, y=100.0) -> (x*y=→"AIR TEMPERATURE  Calibration Error":dbl)
        n1855 = property on="Language Selection" class="Enum (strict)"("Visible"=w2484) -> ()  [unwired: 2 in, 2 out]
        n1856 = property on="Tab Control 7" class="TabCtl (strict)"("Disabled"=w2485) -> ()  [unwired: 2 in, 2 out]
        n1857 = property on="AIR TEMP INTERCEPT:" class="DigNum (strict)"("Disabled"=w2485) -> ()  [unwired: 2 in, 2 out]
        n1858 = property on="CH-POWER -" class="DigNum (strict)"("Disabled"=w2485) -> ()  [unwired: 2 in, 2 out]
        n1859 = property on="CH-POWER +" class="DigNum (strict)"("Disabled"=w2485) -> ()  [unwired: 2 in, 2 out]
        n1860 = property on="AIR TEMPERATURE :" class="DigNum (strict)"("Disabled"=w2485) -> ()  [unwired: 2 in, 2 out]
        n1861 = property on="STROKE GAIN :" class="DigNum (strict)"("Disabled"=w2485) -> ()  [unwired: 2 in, 2 out]
        n1862 = property on="SPEED OUT:" class="DigNum (strict)"("Disabled"=w2485) -> ()  [unwired: 2 in, 2 out]
        n1863 = property on="CH-HUMIDITY DRY" class="DigNum (strict)"("Disabled"=w2485) -> ()  [unwired: 2 in, 2 out]
        n1864 = property on="HUMIDITY:" class="DigNum (strict)"("Disabled"=w2485) -> ()  [unwired: 2 in, 2 out]
        n1865 = property on="CH-HUMIDITY WET" class="DigNum (strict)"("Disabled"=w2485) -> ()  [unwired: 2 in, 2 out]
        n1866 = property on="TEMPERATURE :" class="DigNum (strict)"("Disabled"=w2485) -> ()  [unwired: 2 in, 2 out]
        n1867 = property on="DISPLACEMENT :" class="DigNum (strict)"("Disabled"=w2485) -> ()  [unwired: 2 in, 2 out]
        n1868 = property on="CH-HEATER" class="DigNum (strict)"("Disabled"=w2485) -> ()  [unwired: 2 in, 2 out]
        n1869 = property on="TEMP INTERCEPT:" class="DigNum (strict)"("Disabled"=w2485) -> ()  [unwired: 2 in, 2 out]
        n1870 = property on="FRIC. FORCE :" class="DigNum (strict)"("Disabled"=w2485) -> ()  [unwired: 2 in, 2 out]
      }
    }
    n1871 = local read "RUN"() -> (w1879:bool)
    n1872 = local read "RUN"() -> (w1877:bool)
    n1873 = disable-structure shown="Disabled" {
      disable-tunnel: [w1894 _] -> w1860
      disable-tunnel: [w1893 _] -> w1858
      frame Disabled {
        n1874 = local read "Temperature before test"() -> (w1887:dbl)
        n1875 = local read "Temperature after test"() -> (w1900:dbl)
        n1876 = case shown="True" "Save Results" {
          frame False {
          }
          frame True {
            w1916 = "\r"
            n1877 = local write "Save Results"(FALSE ("OK Button 5")) -> ()
            n1878 = local read "Temperature before test"() -> (w1954:dbl)
            n1879 = local read "Temperature after test"() -> (w1956:dbl)
            n1880 = local read "Humidity before test"() -> (w1953:dbl)
            n1881 = local read "Humidity after test"() -> (w1955:dbl)
            n1882 = local read "WS1.4"() -> (w1960:dbl)
            n1883 = local read "AVP"() -> (w1958:dbl)
            n1884 = Number To Fractional String(number=w1960, width (-)=i16 6, precision (6)=i16 1) -> (F-format string=w1920:string)  [unwired: 1 in]
            n1885 = local read "MWSD"() -> (w1957:dbl)
            n1886 = local read "String"() -> (w1949:string)
            n1887 = local read "FILE"() -> (w1952:string)
            n1888 = local read "HCF"() -> (w1959:dbl)
            n1889 = Number To Fractional String(number=w1953, width (-)=i16 6, precision (6)=i16 1) -> (F-format string=w1945:string)  [unwired: 1 in]
            n1890 = Number To Fractional String(number=w1954, width (-)=i16 6, precision (6)=i16 1) -> (F-format string=w1942:string)  [unwired: 1 in]
            n1891 = Number To Fractional String(number=w1955, width (-)=i16 6, precision (6)=i16 1) -> (F-format string=w1938:string)  [unwired: 1 in]
            n1892 = Number To Fractional String(number=w1956, width (-)=i16 6, precision (6)=i16 1) -> (F-format string=w1934:string)  [unwired: 1 in]
            n1893 = Number To Fractional String(number=w1958, width (-)=i16 6, precision (6)=i16 3) -> (F-format string=w1927:string)  [unwired: 1 in]
            n1894 = Concatenate Strings(w1949, w1952) -> (w1971:string)
            n1895 = Number To Fractional String(number=w1957, width (-)=i16 6, precision (6)=i16 1) -> (F-format string=w1931:string)  [unwired: 1 in]
            n1896 = Number To Fractional String(number=w1959, width (-)=i16 6, precision (6)=i16 2) -> (F-format string=w1925:string)  [unwired: 1 in]
            n1897 = Concatenate Strings("(" ("string"), w1920, ")Microns" ("string")) -> (w1919:string)
            n1898 = local read "REMARKS"() -> (w1951:string)
            "REMARKS 2" <- w1951
            n1899 = Concatenate Strings("(" ("string"), w1945, " ) % RH," ("string")) -> (w1946:string)
            n1900 = Concatenate Strings(w1925, ")" ("string")) -> (w1923:string)
            n1901 = Concatenate Strings("(" ("string"), w1942, ")  Deg C ," ("string")) -> (w1941:string)
            n1902 = Concatenate Strings("(" ("string"), w1938, " ) % RH," ("string")) -> (w1937:string)
            n1903 = Concatenate Strings("(" ("string"), w1934, ")  Deg C ," ("string")) -> (w1933:string)
            n1904 = Concatenate Strings("(" ("string"), w1931, ")  Microns," ("string")) -> (w1930:string)
            n1905 = Concatenate Strings("(" ("string"), w1927, ")  kPa," ("string")) -> (w1917:string)
            n1906 = Concatenate Strings(w1971, ".dwm" ("Substring")) -> (w1969:string)
            n1907 = String To Path(string=w1969) -> (path=w1968:path)
            n1908 = Concatenate Strings(w1951, w1916, " Humidity before test= " ("Substring"), w1946, w1916, " Temperature before test = " ("Substring"), w1941, w1916, " Humidity after test= " ("Substring"), w1937, w1916, "Temperature after test = " ("Substring"), w1933, w1916, "MSD = " ("Substring"), w1930, w1916, "  AVP = " ("Substring"), w1917, w1916, "  HCF                     =( " ("Substring"), w1923, w1916, " WS1.4                  = " ("Substring"), w1919, w1916) -> (w1915:string)
            "data" <- w1915
            n1909 = call <vilib>:"Write Characters To File.vi"("append to file? (new file:F)"=FALSE, "character string"=w1915, "file path (dialog if empty)"=w1968) -> ()  [unwired: 2 in, 1 out]
            n1910 = Match Pattern(string=w1915, regular expression="!") -> (after substring=→"export":string)  [unwired: 1 in, 3 out]
          }
        }
        n1911 = Add(x=231.864, y=w1887) -> (x+y=w1884:dbl)
        n1912 = Add(x=231.864, y=w1900) -> (x+y=w1897:dbl)
        n1913 = Divide(x=1705.984, y=w1884) -> (x/y=w1885:dbl)
        n1914 = Divide(x=1705.984, y=w1897) -> (x/y=w1898:dbl)
        n1915 = local read "Humidity before test"() -> (w1889:dbl)
        n1916 = local read "Humidity after test"() -> (w1902:dbl)
        n1917 = Subtract(x=8.017352 ("y"), y=w1885) -> (x-y=w1911:dbl)
        n1918 = Subtract(x=8.017352 ("y"), y=w1898) -> (x-y=w1905:dbl)
        n1919 = expression code="10**y"(w1911) -> (w1891:dbl)
        n1920 = expression code="10**y"(w1905) -> (w1904:dbl)
        n1921 = Multiply(x=w1889, y=w1891) -> (x*y=w1890:dbl)
        n1922 = Multiply(x=w1902, y=w1904) -> (x*y=w1903:dbl)
        n1923 = Divide(x=w1890, y=750.0) -> (x/y=w1906:dbl)
        n1924 = Divide(x=w1903, y=750.0) -> (x/y=w1907:dbl)
        n1925 = Add(x=w1906, y=w1907) -> (x+y=w1908:dbl)
        n1926 = Divide(x=w1908, y=2.0) -> (x/y=w1910:dbl)
        n1927 = local write "AVP"(w1910) -> ()
        n1928 = Subtract(x=1.4, y=w1910) -> (x-y=w1893:dbl)
        n1929 = local read "HCF"() -> (w1894:dbl)
      }
      frame Enabled {
      }
    }
    n1930 = case shown="True" "EDIT 3" {
      frame False {
      }
      frame True {
        n1931 = local write "EDIT 3"(FALSE ("EDIT 3")) -> ()
        n1932 = local write "Main Tab"(T2."About" ("Main Tab")) -> ()
      }
    }
    n1933 = case shown="False" w1879 {
      frame False {
        n1934 = local read "stopT"() -> (w2857:bool)
        n1935 = case shown="True" w2857 {
          frame False {
          }
          frame True {
            n1936 = local write "stopT"(FALSE) -> ()
          }
        }
      }
      frame True {
        "stopT" <- TRUE
      }
    }
    n1937 = case shown="False" w1877 {
      frame False {
      }
      frame True {
      }
    }
    n1938 = case shown="True" w1867 {
      frame False {
        n1939 = property on="Password 2" class="Str"("Visible"=FALSE) -> ()  [unwired: 2 in, 2 out]
        n1940 = local write "Password 2"("" ("Password")) -> ()
      }
      frame True {
        n1941 = property on="Password 2" class="Str"("Visible"=TRUE) -> ()  [unwired: 2 in, 2 out]
        n1942 = Equal?(x="Password 2", y="HFRR1234") -> (x = y?=w1999:bool)
        n1943 = case shown="True" w1999 {
          tunnel: "Password 2" -> [w2002 _]
          frame False {
            n1944 = String Length(string=w2002) -> (length=w2003:i32)
            n1945 = Greater Than 0?(x=w2003) -> (x > 0?=w2001:bool)
            n1946 = case shown="False" w2001 {
              frame False {
                n1947 = property on="Password 2" class="Str"("Caption.Text"="Password (Advance Setting)") -> ()  [unwired: 2 in, 2 out]
              }
              frame True {
                n1948 = property on="Password 2" class="Str"("Caption.Text"="Incorrect Password!") -> ()  [unwired: 2 in, 2 out]
              }
            }
          }
          frame True {
            n1949 = local write "EDIT 2"(FALSE ("EDIT 2")) -> ()
            n1950 = local write "Password 2"("" ("Password")) -> ()
            n1951 = local write "Main Tab"(T2."Advance" ("Main Tab")) -> ()
            n1952 = local write "Main Dashboard Buttons"(T1."Advance" ("Main Dashboard Buttons")) -> ()
          }
        }
      }
    }
    n1953 = case shown="True" "Prog Uno" {
      frame False {
      }
      frame True {
        n1954 = stacked-sequence {
          frame #0 {
            n1955 = Delete(path (use dialog)=path "C:/LAB-IQ-NXT/UNOCOMPILE.bat" ("working directory")) -> ()  [unwired: 4 in, 3 out]
          }
          frame #1 {
            n1956 = local read "Com Port 1"() -> (w2464:refnum<visa-resource-name>)
            n1957 = Concatenate Strings("cmd.exe /c \"mode " ("command line"), w2464, ":1200,n,8,1\"\n" ("command line")) -> (w2469:string)
            n1958 = Concatenate Strings(w2469, "CD\\\nCD WinDucom\navrdude -C avrdude.conf -v -patmega328p -carduino -P" ("command line"), w2464, " -b115200 -D -Uflash:w:UNO_V20.hex:i\n" ("command line"), "\r") -> (w2471:string)
            "STR" <- w2471
            n1959 = call <vilib>:"Write Characters To File.vi"("append to file? (new file:F)"=FALSE, "character string"=w2471, "file path (dialog if empty)"=path "C:/LAB-IQ/UNOCOMPILE.bat" ("working directory")) -> ()  [unwired: 2 in, 1 out]
          }
          frame #2 {
            n1960 = disable-structure shown="Disabled" {
              frame Disabled {
                w2475 = "cmd.exe  /c \"C:\\LAB-IQ-NXT\\UNOCOMPILE.bat\"" ("string")
                n1961 = local write "Prog Uno"(FALSE ("run minimized? (F)")) -> ()
                n1962 = call <vilib>:"System Exec.vi"("expected output size  (4096)"=u32 65535, "run minimized? (F)"=FALSE, "wait until completion? (T)"=TRUE ("run minimized? (F)"), "working directory"=path "C:/LAB-IQ-NXT", "standard input"=w2475, "command line"=w2475) -> ("error out"=w2474:errorcluster, "standard output"=→"String 42":string)  [unwired: 2 in, 2 out]
                "error out 3" <- w2474
                n1963 = flat-sequence {
                  tunnel: w2474 -> [_]
                  frame #0 {
                  }
                }
              }
              frame Enabled {
              }
            }
          }
        }
      }
    }
    n1964 = case shown="\"ISO 12156\"" "TEST STANDARD" {
      tunnel: [2.0 ("Set Temp") 0.0 ("Set Temp") 2.0 ("Set Temp") 0.0 ("Set Temp")] -> w1868
      frame "ASTM D6079", Default {
        w2421 = 50.0 ("Hz")
        w2422 = 53.0 ("Set Rh")
        w2424 = 1.0 ("Set Strk")
        w2423 = 60.0 ("Set Temp")
        # "astm hide"
        n1965 = local write "NORMAL LOAD"(200.0 ("NORMAL LOAD")) -> ()
        n1966 = local write "Set Strk"(w2424) -> ()
        n1967 = local write "Set Hz"(w2421) -> ()
        n1968 = local write "Set Temp"(w2423) -> ()
        n1969 = local write "Set Rh"(w2422) -> ()
        n1970 = local write "test time"(75.0 ("test time")) -> ()
        n1971 = local write "Set Stroke:"(w2424) -> ()
        n1972 = local write "Set Humidity:"(w2422) -> ()
        n1973 = local write "Set Frequency:"(w2421) -> ()
        n1974 = local write "Set Temperature:"(w2423) -> ()
        "Test Standard" <- "ASTM D6079" ("Test Standard 2")
      }
      frame "ISO 12156" {
        n1975 = local write "Set Strk"(1.0 ("Set Strk")) -> ()
        n1976 = local write "NORMAL LOAD"(200.0 ("NORMAL LOAD")) -> ()
        n1977 = local write "Set Temp"(60.0 ("Set Temp")) -> ()
        n1978 = local write "test time"(75.0 ("test time")) -> ()
        n1979 = local write "Set Hz"(50.0 ("Hz")) -> ()
        n1980 = local write "Set Rh"(53.0 ("Set Rh")) -> ()
      }
      frame "CEC F-096-A-06" {
        n1981 = local write "Set Strk"(1.0 ("Set Strk")) -> ()
        n1982 = local write "NORMAL LOAD"(200.0 ("NORMAL LOAD")) -> ()
        n1983 = local write "Set Temp"(60.0 ("Set Temp")) -> ()
        n1984 = local write "test time"(75.0 ("test time")) -> ()
        n1985 = local write "Set Hz"(50.0 ("Hz")) -> ()
        n1986 = local write "Set Rh"(53.0 ("Set Rh")) -> ()
      }
      frame "Custom" {
      }
    }
    n1987 = case shown="True" "Prog Due" {
      frame False {
      }
      frame True {
        n1988 = stacked-sequence {
          frame #0 {
            n1989 = Delete(path (use dialog)=path "C:/LAB-IQ/DUECOMPILE.bat" ("working directory")) -> ()  [unwired: 4 in, 3 out]
          }
          frame #1 {
            n1990 = disable-structure shown="Disabled" {
              frame Disabled {
                n1991 = local read "visa due"() -> (w2446:string)
                n1992 = Concatenate Strings("cmd.exe /c \"mode " ("command line"), w2446, ":1200,n,8,1\"\n" ("command line")) -> (w2451:string)
                n1993 = Concatenate Strings(w2451, "CD\\\nCD WinDucom\nTIMEOUT 1\n bossac.exe -i -d --port=" ("command line"), w2446, " -U false -e -w -v -b DUE.bin -R\n" ("command line"), "\r") -> (w2453:string)
                "concatenated string 2" <- w2453
                n1994 = call <vilib>:"Write Characters To File.vi"("append to file? (new file:F)"=FALSE, "character string"=w2453, "file path (dialog if empty)"=path "C:/LAB-IQ-NXT/DUECOMPILE.bat" ("working directory")) -> ()  [unwired: 2 in, 1 out]
              }
              frame Enabled {
              }
            }
          }
          frame #2 {
            # "C:\\LAB-IQ-NXT\\DUECOMPILE.bat"
            n1995 = disable-structure shown="Disabled" {
              frame Disabled {
                w2458 = "cmd.exe  /c \"C:\\LAB-IQ-NXT\\DUECOMPILE.bat\"" ("string")
                n1996 = call <vilib>:"System Exec.vi"("expected output size  (4096)"=u32 65535, "run minimized? (F)"=FALSE, "wait until completion? (T)"=TRUE ("run minimized? (F)"), "working directory"=path "C:/LAB-IQ-NXT", "standard input"=w2458, "command line"=w2458) -> ("error out"=w2457:errorcluster, "standard output"=→"String 44":string)  [unwired: 2 in, 2 out]
                "error out 4" <- w2457
                n1997 = flat-sequence {
                  tunnel: w2457 -> [_]
                  frame #0 {
                  }
                }
              }
              frame Enabled {
              }
            }
            n1998 = local write "Prog Due"(FALSE ("Prog Due")) -> ()
          }
        }
      }
    }
    n1999 = Or(x=w1865, y=w1863) -> (x .or. y?=w1864:bool)
    n2000 = case shown="\"About\"" w1862 {
      tunnel: [T27."Acquire" ("Main Tab") T27."Compare Files" ("Main Tab") T27."About" ("Main Tab")] -> w1875
      frame "Acquire", Default {
      }
      frame "Compare Files" {
      }
      frame "About" {
      }
    }
    n2001 = Or(x=w1869, y="OPEN") -> (x .or. y?=w1870:bool)
    n2002 = case shown="True" w1870 {
      tunnel: w1869 -> [_ w2010]
      frame False {
      }
      frame True {
        n2003 = stacked-sequence {
          tunnel: w2010 -> [_ w2077 _ _]
          frame #0 {
            w2026 = "  " ("String 6")
            n2004 = local write "OPEN"(FALSE ("open")) -> ()
            n2005 = local read "string1 2"() -> (w2014:string)
            n2006 = local read "string1 3"() -> (w2013:string)
            n2007 = local read "string1 4"() -> (w2012:string)
            n2008 = property on="OPEN" class="Bool (strict)"("Visible"=FALSE) -> ()  [unwired: 2 in, 2 out]
            n2009 = local write "String 6"(w2026) -> ()
            n2010 = local write "String 7"(w2026) -> ()
            n2011 = local write "String 8"(w2026) -> ()
            n2012 = local write "String 12"(w2026) -> ()
            n2013 = local read "OK Button 16"() -> (w2011:bool)
            n2014 = String To Path(string=w2014) -> (path=w2022:path)
            n2015 = String To Path(string=w2013) -> (path=w2021:path)
            n2016 = String To Path(string=w2012) -> (path=w2020:path)
            n2017 = case shown="True" w2011 {
              tunnel: [w2027 w2028] -> w2015
              frame False {
                n2018 = local read "string1"() -> (w2027:string)
              }
              frame True {
                n2019 = local read "String Indicator 4"() -> (w2028:string)
              }
            }
            n2020 = Open/Create/Replace File "Open File"(file path (use dialog)=w2022) -> (refnum out=w2018:refnum<file>)  [unwired: 5 in, 2 out]
            n2021 = Open/Create/Replace File "Open File"(file path (use dialog)=w2021) -> (refnum out=w2017:refnum<file>)  [unwired: 5 in, 2 out]
            n2022 = Open/Create/Replace File "Open File"(file path (use dialog)=w2020) -> (refnum out=w2016:refnum<file>)  [unwired: 5 in, 2 out]
            n2023 = while {
              tunnel: w2018 -> [w2040]
              i -> [w2036]
              stop <- w2035 continue-if-true
              (unwired) TRUE ("line mode (F)")
              n2024 = Read from Text File "Read File"(file (use dialog)=w2040) -> (text=w2037:string)  [unwired: 3 in, 3 out]
              n2025 = local write "Numeric 11"(w2036) -> ()
              n2026 = String Length(string=w2037) -> (length=w2039:i32)
              n2027 = Greater?(x=w2039, y=1) -> (0:w2035:bool)
            }
            n2028 = while {
              tunnel: w2017 -> [w2046]
              i -> [w2042]
              stop <- w2041 continue-if-true
              (unwired) TRUE ("line mode (F)")
              n2029 = Read from Text File "Read File"(file (use dialog)=w2046) -> (text=w2043:string)  [unwired: 3 in, 3 out]
              n2030 = local write "Numeric 12"(w2042) -> ()
              n2031 = String Length(string=w2043) -> (length=w2045:i32)
              n2032 = Greater?(x=w2045, y=1) -> (0:w2041:bool)
            }
            n2033 = while {
              tunnel: w2016 -> [w2052]
              i -> [w2048]
              stop <- w2047 continue-if-true
              (unwired) TRUE ("line mode (F)")
              n2034 = Read from Text File "Read File"(file (use dialog)=w2052) -> (text=w2049:string)  [unwired: 3 in, 3 out]
              n2035 = local write "Numeric 13"(w2048) -> ()
              n2036 = String Length(string=w2049) -> (length=w2051:i32)
              n2037 = Greater?(x=w2051, y=1) -> (0:w2047:bool)
            }
            n2038 = String To Path(string=w2015) -> (path=w2023:path)
            n2039 = Open/Create/Replace File "Open File"(file path (use dialog)=w2023) -> (refnum out=w2019:refnum<file>)  [unwired: 5 in, 2 out]
            n2040 = while {
